vi "Convert Mouse Motion Event Data.vi"(11 "Event Data":u8[](array[numeric])) -> (3 "Mouse Motion Event":T1)   [LabVIEW 2014, in "LibSDL2.lvlib"]
uses:
  LibSDL2.lvlib
  Controls/Mouse Motion Event.ctl
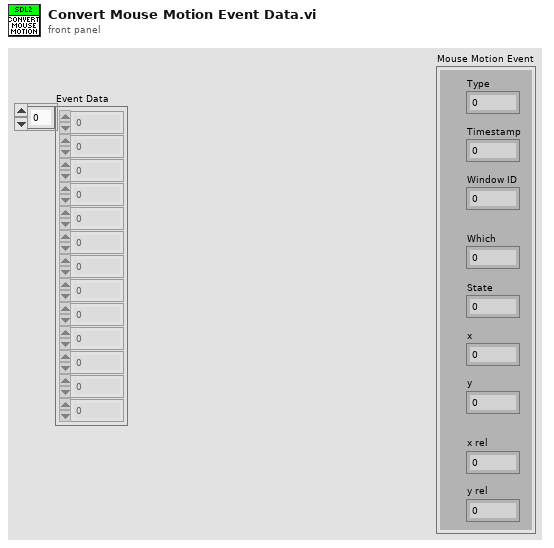
[diagram p1: front panel]
types:
  T1 = typedef "LibSDL2.lvlib/Mouse Motion Event.ctl" = cluster{"Type":u32, "Timestamp":u32, "Window ID":u32, "Which":u32, "State":u32, "x":i32, "y":i32, "x rel":i32, "y rel":i32}
  T2 = cluster{"[0]":u32, "[1]":u32, "[2]":u32, "[3]":u32, "[4]":u32, "[5]":u32, "[6]":u32, "[7]":u32, "[8]":u32}
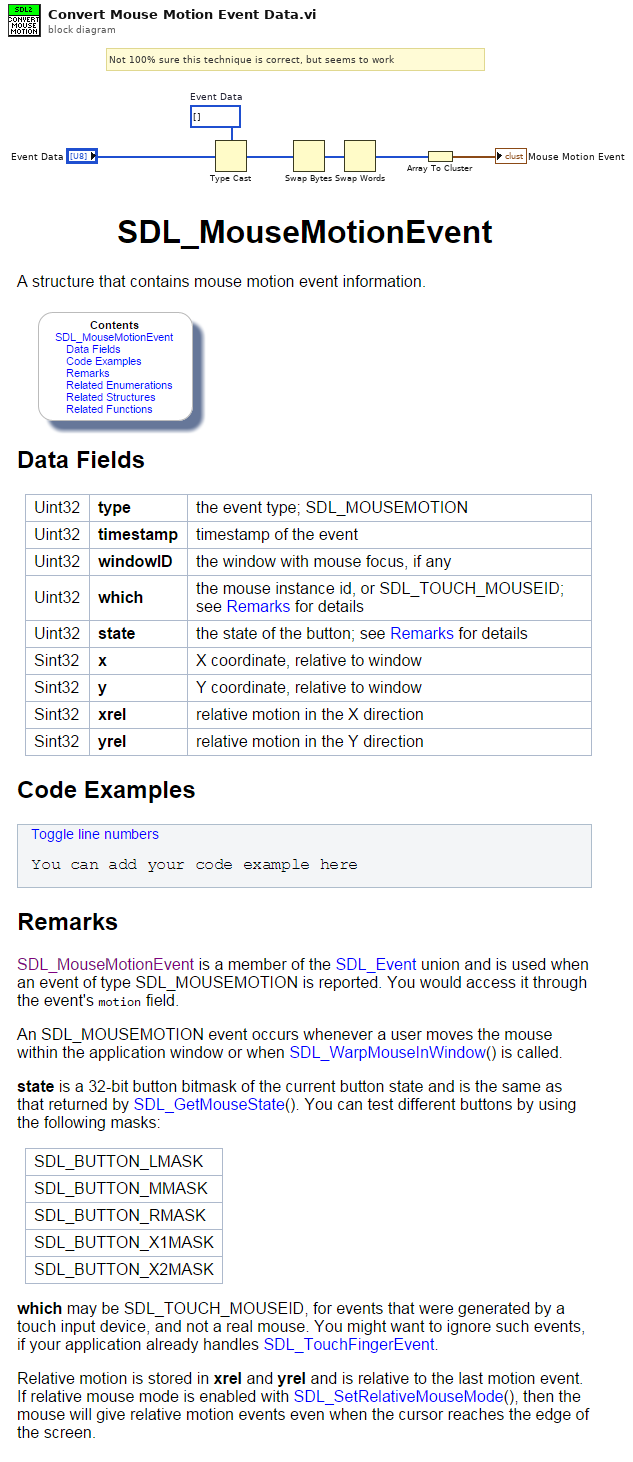
[diagram p0: block diagram]
diagram:
  w6 = u32[] []  # Event Data
  # "Not 100% sure this technique is correct, but seems to work"
  n1 = Type Cast(type=w6, x="Event Data") -> (*(type *) &x=w3:u32[])
  n2 = Swap Bytes(anything=w3) -> (byte swapped=w4:u32[])
  n3 = Swap Words(1:w4) -> (0:w2:u32[])
  n4 = Array To Cluster(array=w2) -> (cluster=→"Mouse Motion Event":T2)
